vi "Scale Speed to PWM.vi"(8 "Error In":errorcluster, 9 "Move Constraints":T1={"Velocity Profile Type"=enum."S Curve", "Max Velocity"=2.0, "Max Acceleration"=1.0, "Max Deceleration"=1.0, "Max Jerk"=2.0, "Initial Velocity"=0.0, "Final Velocity"=0.0} {"Final Velocity" format="%#.6g"; "Initial Velocity" format="%#.6g"; "Max Jerk" format="%#.6g"; "Max Deceleration" format="%#.6g"; "Max Acceleration" format="%#.6g"; "Max Velocity" format="%#.6g"}, 10 "Desired Speed (in/s)":dbl) -> (0 "Error Out":errorcluster, 2 "Motor Duty Cycle":dbl)   [LabVIEW 2013]
doc: "This sub-VI scales the desired command speed to the motor into a PWM duty cycle. Tests need to be run\nto determine the deadband of the motor, and motor velocity constant for linear scaling. Nonlinear scaling\ncould be set up as well."
uses:
  <vilib>/MotionAssistant/MotionAssistant.llb/Move Constraints.ctl
  <vilib>/MotionAssistant/MotionAssistant.llb/Velocity Profile Type Enum.ctl
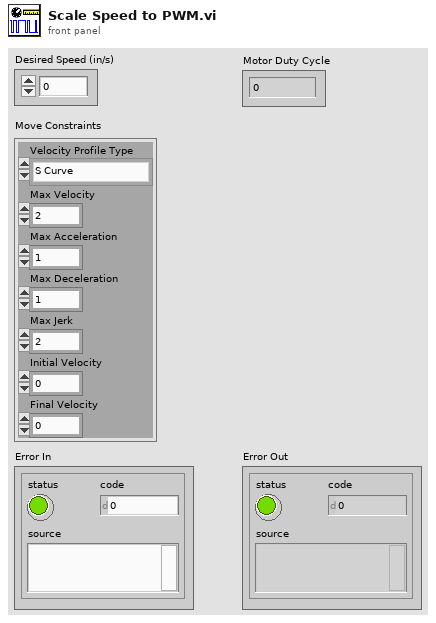
[diagram p1: front panel]
types:
  T1 = typedef "Move Constraints.ctl" = cluster{"Velocity Profile Type":T2, "Max Velocity":dbl, "Max Acceleration":dbl, "Max Deceleration":dbl, "Max Jerk":dbl, "Initial Velocity":dbl, "Final Velocity":dbl}
  T2 = typedef "Velocity Profile Type Enum.ctl" = enum32{"Trapezoidal", "S Curve"}
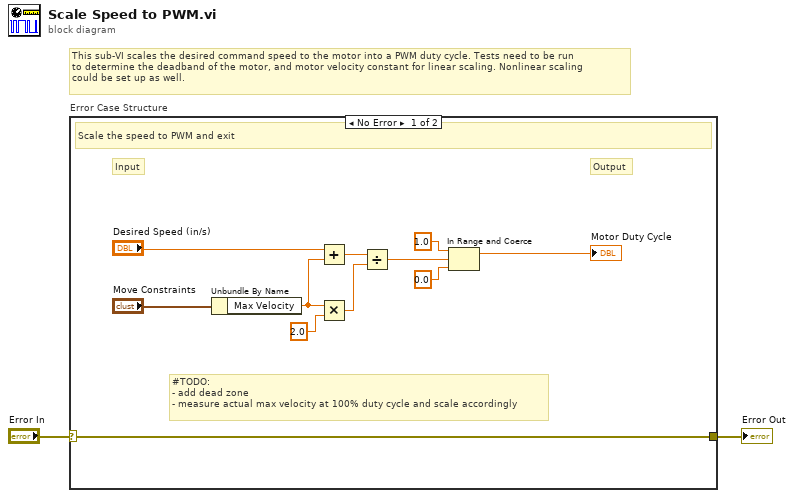
[diagram p0: block diagram]
diagram:
  # "This sub-VI scales the desired command speed to the motor into a PWM duty cycle. Tests need to be run\nto determine the deadband of the motor, and motor velocity constant for linear scaling. Nonlinear scaling\ncould be set up as well."
  n1 = case "Error Case Structure" shown="No Error" "Error In" {
    selector: "Error In" -> [w3 w14]
    tunnel: [w3 w14] -> w1
    frame No Error {
      # "#TODO:\n- add dead zone\n- measure actual max velocity at 100% duty cycle and scale accordingly"
      # "Output"
      # "Input"
      # "Scale the speed to PWM and exit"
      n2 = Unbundle By Name("Move Constraints") -> ("Max Velocity"=w10:dbl)
      n3 = Add(x="Desired Speed (in/s)", y=w10) -> (x+y=w11:dbl)
      n4 = Multiply(x=w10, y=2.0) -> (x*y=w8:dbl)
      n5 = Divide(x=w11, y=w8) -> (x/y=w7:dbl)
      n6 = In Range and Coerce(upper limit=1.0, x=w7, lower limit=0.0) -> (coerced(x)=→"Motor Duty Cycle":dbl)  [unwired: 1 out]
    }
    frame Error {
      # "Pass through and exit"
    }
  }
  "Error Out" <- w1
